vi "XY Dialog - Update Y Plots.vi"(8 "error in (no error)":errorcluster, 10 "Tree Selected Paths":string[][](array[string]), 11 "Y Channel Listbox":refnum<vi>) -> (0 "error out":errorcluster)   [LabVIEW 2013, in "Workspace MultiY Graph.lvlib"]
uses:
  Workspace MultiY Graph.lvlib
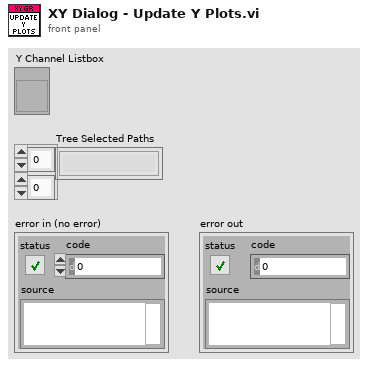
[diagram p1: front panel]
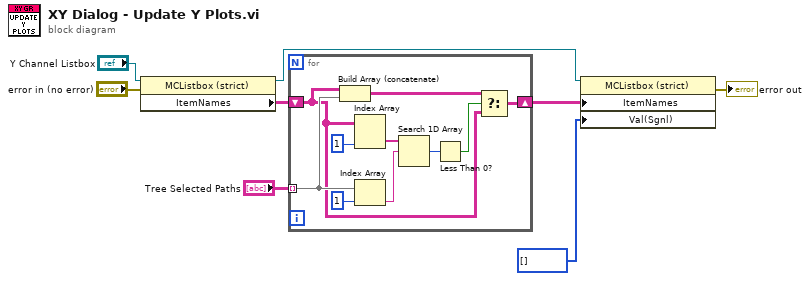
[diagram p0: block diagram]
diagram:
  n1 = property class="MCListbox (strict)"(reference="Y Channel Listbox", error in="error in (no error)") -> (reference out=w4:refnum<vi>, "ItemNames"=w7:string[][])  [unwired: 1 out]
  n2 = for {
    tunnel: "Tree Selected Paths" -> [w12] mode=indexing
    shift-right: [w10] -> w8
    shift-left: w7 -> [w9]
    n3 = Build Array (concatenate)(w9, w12) -> (w11:string[][])
    n4 = Index Array(array=w9, index (col)=1 ("disabled index (col)")) -> (element=w17:string[])  [unwired: 1 in]
    n5 = Index Array(array=w12, index=1) -> (element=w15:string)
    n6 = Search 1D Array(1D array=w17, element=w15) -> (index of element=w14:i32)  [unwired: 1 in]
    n7 = Less Than 0?(x=w14) -> (x < 0?=w13:bool)
    n8 = Select(t=w11, s=w13, f=w9) -> (s? t:f=w10:string[][])
  }
  n9 = property class="MCListbox (strict)"(reference=w4, "ItemNames"=w8, "Val(Sgnl)"=i32[] [] ("Value (Signaling)")) -> (error out=→"error out":errorcluster)  [unwired: 1 in, 1 out]
